vi "seven segment led.vi"(6 "Numeric":dbl, 8 "D":bool, 9 "C":bool, 10 "B":bool, 11 "A":bool) -> (0 "Segment 'f'":bool, 1 "Segment 'e'":bool, 2 "Segment 'd'":bool, 3 "Segment 'c'":bool, 4 "Segment 'b'":bool, 5 "Segment 'g'":bool, 7 "Segment 'a'":bool)   [LabVIEW 2018]
panel:
  # "BINARY INPUTS"
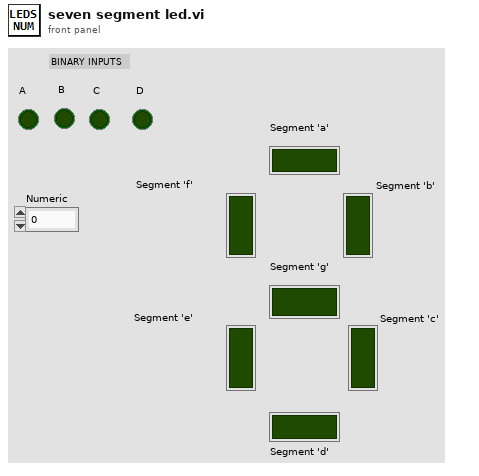
[diagram p1: front panel]
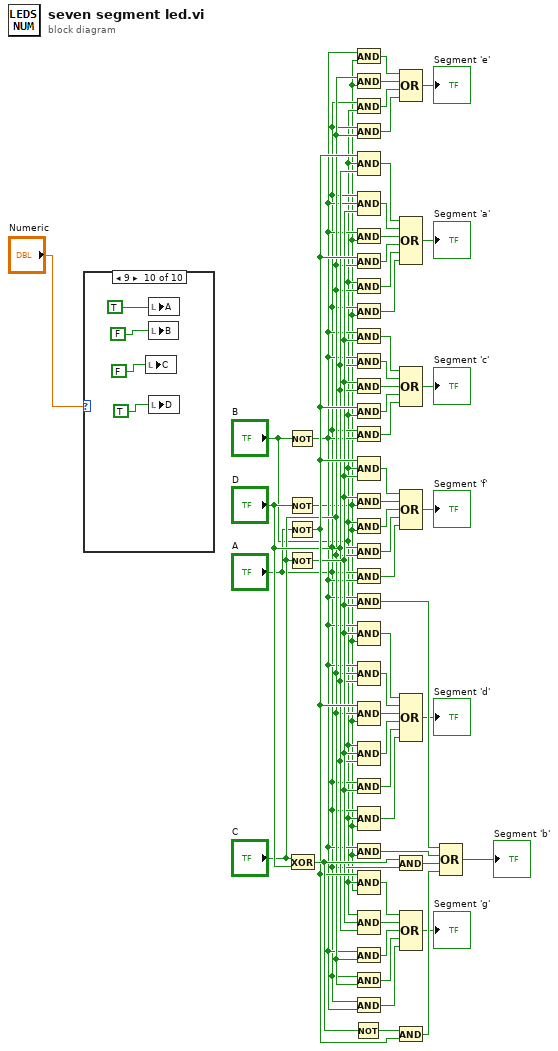
[diagram p0: block diagram]
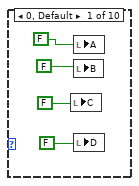
[diagram p2: hidden frame]
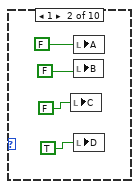
[diagram p3: hidden frame]
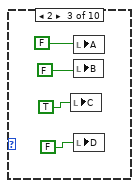
[diagram p4: hidden frame]
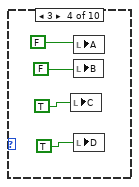
[diagram p5: hidden frame]
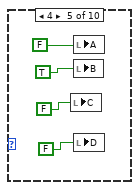
[diagram p6: hidden frame]
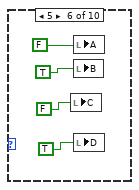
[diagram p7: hidden frame]
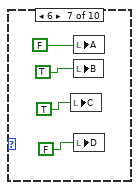
[diagram p8: hidden frame]
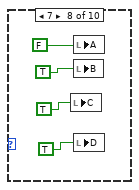
[diagram p9: hidden frame]
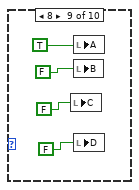
[diagram p10: hidden frame]
diagram:
  n1 = case shown="9" "Numeric" {
    frame 0, Default {
      n2 = local write "C"(FALSE) -> ()
      n3 = local write "A"(FALSE) -> ()
      n4 = local write "B"(FALSE) -> ()
      n5 = local write "D"(FALSE) -> ()
    }
    frame 1 {
      n6 = local write "C"(FALSE) -> ()
      n7 = local write "A"(FALSE) -> ()
      n8 = local write "B"(FALSE) -> ()
      n9 = local write "D"(TRUE) -> ()
    }
    frame 2 {
      n10 = local write "C"(TRUE) -> ()
      n11 = local write "A"(FALSE) -> ()
      n12 = local write "B"(FALSE) -> ()
      n13 = local write "D"(FALSE) -> ()
    }
    frame 3 {
      n14 = local write "C"(TRUE) -> ()
      n15 = local write "A"(FALSE) -> ()
      n16 = local write "B"(FALSE) -> ()
      n17 = local write "D"(TRUE) -> ()
    }
    frame 4 {
      n18 = local write "C"(FALSE) -> ()
      n19 = local write "A"(FALSE) -> ()
      n20 = local write "B"(TRUE) -> ()
      n21 = local write "D"(FALSE) -> ()
    }
    frame 5 {
      n22 = local write "C"(FALSE) -> ()
      n23 = local write "A"(FALSE) -> ()
      n24 = local write "B"(TRUE) -> ()
      n25 = local write "D"(TRUE) -> ()
    }
    frame 6 {
      n26 = local write "C"(TRUE) -> ()
      n27 = local write "A"(FALSE) -> ()
      n28 = local write "B"(TRUE) -> ()
      n29 = local write "D"(FALSE) -> ()
    }
    frame 7 {
      n30 = local write "C"(TRUE) -> ()
      n31 = local write "A"(FALSE) -> ()
      n32 = local write "B"(TRUE) -> ()
      n33 = local write "D"(TRUE) -> ()
    }
    frame 8 {
      n34 = local write "C"(FALSE) -> ()
      n35 = local write "A"(TRUE) -> ()
      n36 = local write "B"(FALSE) -> ()
      n37 = local write "D"(FALSE) -> ()
    }
    frame 9 {
      n38 = local write "C"(FALSE) -> ()
      n39 = local write "A"(TRUE) -> ()
      n40 = local write "B"(FALSE) -> ()
      n41 = local write "D"(TRUE) -> ()
    }
  }
  n42 = Not(x="B") -> (.not. x?=w7:bool)
  n43 = Not(x="D") -> (.not. x?=w2:bool)
  n44 = Not(x="A") -> (.not. x?=w15:bool)
  n45 = Not(x="C") -> (.not. x?=w13:bool)
  n46 = Exclusive Or(1:"D", 2:"C") -> (0:w41:bool)
  n47 = Not(x=w41) -> (.not. x?=w42:bool)
  n48 = And(x=w7, y=w2) -> (x .and. y?=w27:bool)
  n49 = And(x="C", y=w2) -> (x .and. y?=w26:bool)
  n50 = And(x="A", y="B") -> (x .and. y?=w25:bool)
  n51 = And(x="A", y="C") -> (x .and. y?=w24:bool)
  n52 = And(x=w7, y=w2) -> (x .and. y?=w50:bool)
  n53 = And(x=w15, y="C") -> (x .and. y?=w49:bool)
  n54 = And(x="B", y="C") -> (x .and. y?=w48:bool)
  n55 = And(x="A", y=w2) -> (x .and. y?=w47:bool)
  n56 = And(x=w7, y=w13) -> (x .and. y?=w38:bool)
  n57 = And(x=w7, y="D") -> (x .and. y?=w37:bool)
  n58 = And(x=w13, y="D") -> (x .and. y?=w36:bool)
  n59 = And(x=w15, y="B") -> (x .and. y?=w35:bool)
  n60 = And(x="A", y=w7) -> (x .and. y?=w34:bool)
  n61 = And(x=w13, y=w2) -> (x .and. y?=w20:bool)
  n62 = And(x="B", y=w2) -> (x .and. y?=w19:bool)
  n63 = And(x="A", y="C") -> (x .and. y?=w18:bool)
  n64 = And(x="A", y=w7) -> (x .and. y?=w17:bool)
  n65 = And(x=w7, y=w13) -> (x .and. y?=w45:bool)
  n66 = And(x="A", y=w13) -> (x .and. y?=w28:bool)
  n67 = And(x=w7, y=w2) -> (x .and. y?=w44:bool)
  n68 = And(x=w7, y="C") -> (x .and. y?=w10:bool)
  n69 = And(x="A", y="C") -> (x .and. y?=w8:bool)
  n70 = And(x="A", y=w7) -> (x .and. y?=w6:bool)
  n71 = Compound Arithmetic op=AND(w15, "B", "D") -> (w52:bool)
  n72 = Compound Arithmetic op=AND("A", w7, w13) -> (w51:bool)
  n73 = Compound Arithmetic op=AND(w15, "B", w13) -> (w22:bool)
  n74 = Compound Arithmetic op=AND(w7, w13, w2) -> (w32:bool)
  n75 = Compound Arithmetic op=AND(w7, "C", "D") -> (w31:bool)
  n76 = Compound Arithmetic op=AND(w15, "C", w2) -> (w30:bool)
  n77 = Compound Arithmetic op=AND("B", w13, "D") -> (w29:bool)
  n78 = Compound Arithmetic op=AND("A", "B", w2) -> (w5:bool)
  n79 = Compound Arithmetic op=AND(w15, "B", w2) -> (w14:bool)
  n80 = Compound Arithmetic op=AND("B", w13, "D") -> (w11:bool)
  n81 = And(x=w41, y="A") -> (x .and. y?=w43:bool)
  n82 = And(x=w42, y=w15) -> (x .and. y?=w40:bool)
  n83 = Compound Arithmetic op=OR(w27, w26, w25, w24) -> (→"Segment 'e'":bool)
  n84 = Compound Arithmetic op=OR(w52, w51, w50, w49, w48, w47) -> (→"Segment 'a'":bool)
  n85 = Compound Arithmetic op=OR(w38, w37, w36, w35, w34) -> (→"Segment 'c'":bool)
  n86 = Compound Arithmetic op=OR(w22, w20, w19, w18, w17) -> (→"Segment 'f'":bool)
  n87 = Compound Arithmetic op=OR(w32, w31, w30, w29, w28, w5) -> (→"Segment 'd'":bool)
  n88 = Compound Arithmetic op=OR(w14, w11, w10, w8, w6) -> (→"Segment 'g'":bool)
  n89 = Compound Arithmetic op=OR(w45, w44, w43, w40) -> (→"Segment 'b'":bool)
